vi "prefixConversion.vi"(11 "prefix":u32) -> (3 "Numeric":dbl)   [LabVIEW 2017]
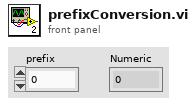
[diagram p1: front panel]
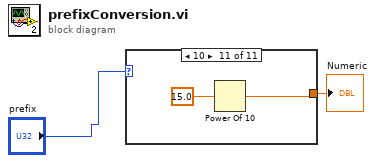
[diagram p0: block diagram]
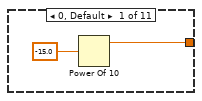
[diagram p2: hidden frame]
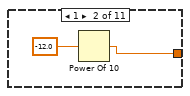
[diagram p3: hidden frame]
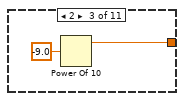
[diagram p4: hidden frame]
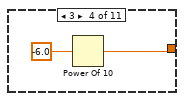
[diagram p5: hidden frame]
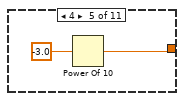
[diagram p6: hidden frame]
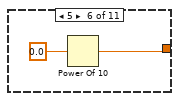
[diagram p7: hidden frame]
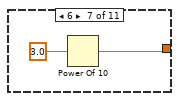
[diagram p8: hidden frame]
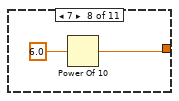
[diagram p9: hidden frame]
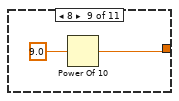
[diagram p10: hidden frame]
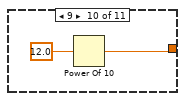
[diagram p11: hidden frame]
diagram:
  n1 = case shown="10" "prefix" {
    tunnel: [w4 w5 w8 w9 w11 w13 w15 w17 w19 w21 w23] -> w2
    frame 0, Default {
      n2 = Power Of 10(x=-15.0) -> (10^x=w4:dbl)
    }
    frame 1 {
      n3 = Power Of 10(x=-12.0) -> (10^x=w5:dbl)
    }
    frame 2 {
      n4 = Power Of 10(x=-9.0) -> (10^x=w8:dbl)
    }
    frame 3 {
      n5 = Power Of 10(x=-6.0) -> (10^x=w9:dbl)
    }
    frame 4 {
      n6 = Power Of 10(x=-3.0) -> (10^x=w11:dbl)
    }
    frame 5 {
      n7 = Power Of 10(x=0.0) -> (10^x=w13:dbl)
    }
    frame 6 {
      n8 = Power Of 10(x=3.0) -> (10^x=w15:dbl)
    }
    frame 7 {
      n9 = Power Of 10(x=6.0) -> (10^x=w17:dbl)
    }
    frame 8 {
      n10 = Power Of 10(x=9.0) -> (10^x=w19:dbl)
    }
    frame 9 {
      n11 = Power Of 10(x=12.0) -> (10^x=w21:dbl)
    }
    frame 10 {
      n12 = Power Of 10(x=15.0) -> (10^x=w23:dbl)
    }
  }
  "Numeric" <- w2
